vi "NF WF1973_74 SYST Err.vi"(0 "VISAsession":refnum<visa-resource-name>, 1 "Error IN":errorcluster) -> (3 "Copy VISA":refnum<visa-resource-name>, 4 "Error Number":string, 5 "Error OUT":errorcluster)   [LabVIEW 2010]
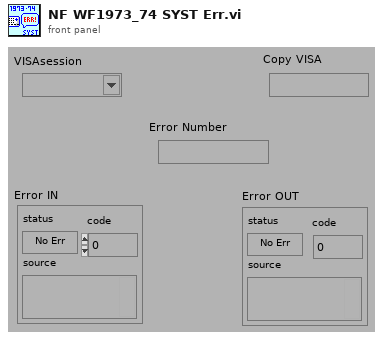
[diagram p1: front panel]
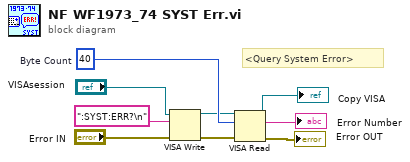
[diagram p0: block diagram]
diagram:
  w9 = u32 40  # Byte Count
  # "<Query System Error>"
  n1 = VISA Write(VISA resource name="VISAsession", write buffer=":SYST:ERR?\n" ("G[â¹ºÏÝÄÞ"), error in (no error)="Error IN") -> (VISA resource name out=w1:refnum<visa-resource-name>, error out=w2:errorcluster)  [unwired: 1 out]
  n2 = VISA Read(VISA resource name=w1, byte count=w9, error in (no error)=w2) -> (VISA resource name out=→"Copy VISA":refnum<visa-resource-name>, read buffer=→"Error Number":string, error out=→"Error OUT":errorcluster)  [unwired: 1 out]
